vi "Write Tag Root.vi"(8 "error in (no error)":errorcluster, 10 "Tag Root":string, 11 "Var_Access in":refnum<class "Bus_Access.lvclass">) -> (0 "error out":errorcluster, 3 "Var_Access out":refnum<class "Bus_Access.lvclass">)   [LabVIEW 2021, in "Bus_Access.lvclass"]
uses:
  Bus_Access.lvclass
  Bus_Access.lvclass/Bus_Access.ctl
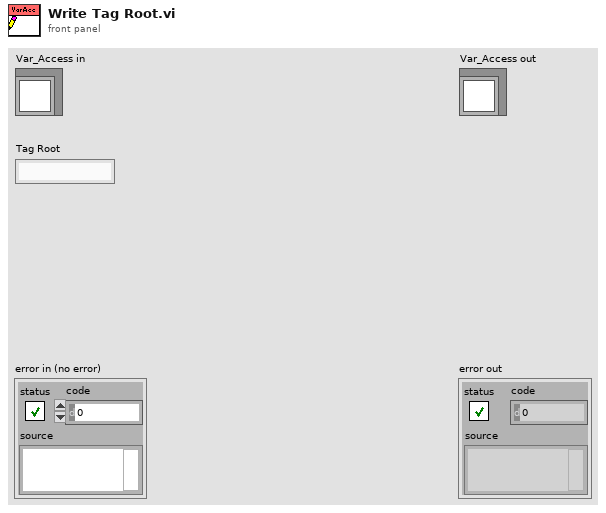
[diagram p1: front panel]
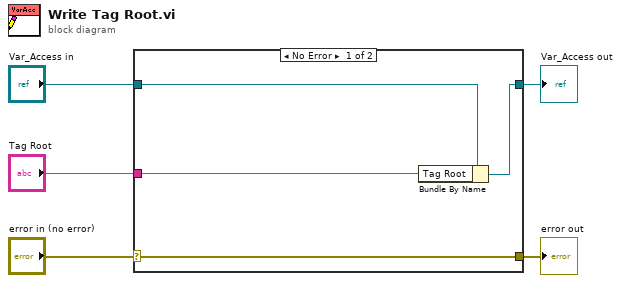
[diagram p0: block diagram]
diagram:
  n1 = case shown="No Error" "error in (no error)" {
    selector: "error in (no error)" -> [w9 w10]
    tunnel: [w9 w10] -> w4
    tunnel: [w7 w11] -> w2
    tunnel: "Var_Access in" -> [w8 w11]
    tunnel: "Tag Root" -> [w6 _]
    frame No Error {
      n2 = Bundle By Name(cluster=w8, "Tag Root"=w6) -> (w7:refnum<class "Bus_Access.lvclass">)
    }
    frame Error {
    }
  }
  "error out" <- w4
  "Var_Access out" <- w2
